vi "Generate multi-line AO sequence.vi"(11 "Variables":T1 {"Dwell time" format="%#_6f"; "Sample Clock Rate" format="%#_6f"}) -> (3 "Pockels modulation sequence":dbl[](array[numeric]))   [LabVIEW 2017]
uses:
  Typedefs/Pockels mod gen variables cluster.ctl
  Typedefs/Imaging Protocols enum.ctl
panel:
  out "Single line (points)":i32
  out "Full sequence (points)":i32
  out "Length of single line (ms)":dbl format="%#_6f"
  out "Length of sequence (ms)":dbl format="%#_6f"
  out "Multi-line pockels modulation waveform":dbl[](graph)
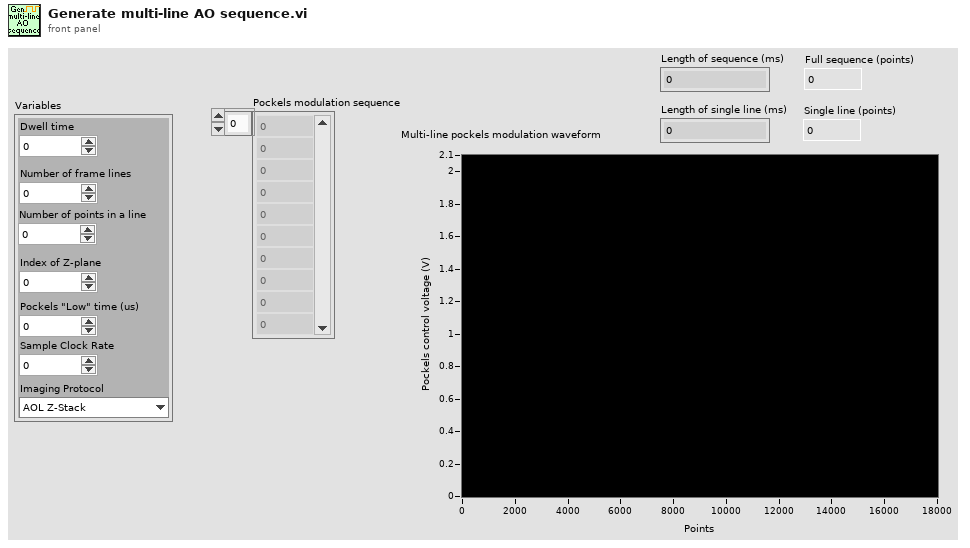
[diagram p1: front panel]
types:
  T1 = typedef "Pockels mod gen variables cluster.ctl" = cluster{"Dwell time":dbl, "Number of frame lines":i32, "Number of points in a line":i32, "Index of Z-plane":i32, "Pockels \"Low\" time (us)":dbl, "Sample Clock Rate":dbl, "Imaging Protocol":T2}
  T2 = typedef "Imaging Protocols enum.ctl" = enum16{"AOL Z-Stack", "Motor Z Stack", "Functional Acquisition", "Single Plane Acquisition", "Volume Acquisition", "Live Imaging", "Live Plane Imaging", "Live Volume Imaging"}
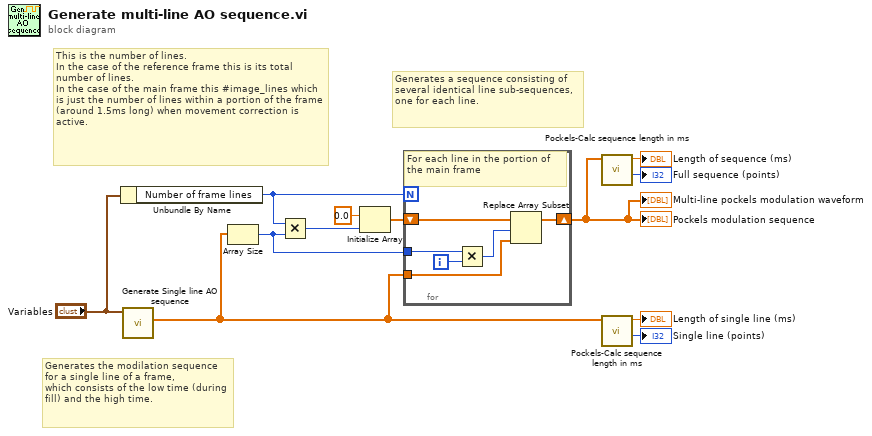
[diagram p0: block diagram]
diagram:
  # "This is the number of lines.\nIn the case of the reference frame this is its total number of lines.\nIn the case of the main frame this #image_lines which is just the number of lines within a portion of the frame (around 1.5ms long) when movement correction is active."
  # "Generates a sequence consisting of several identical line sub-sequences, one for each line."
  # "Generates the modilation sequence for a single line of a frame,\nwhich consists of the low time (during fill) and the high time."
  n1 = Unbundle By Name("Variables") -> ("Number of frame lines"=w8:i32)
  n2 = call "Generate Single line AO sequence.vi"("Variables"="Variables") -> ("Single line AO sequence"=w4:dbl[])  [unwired: 10 in]
  n3 = Array Size(array=w4) -> (size(s)=w12:i32)
  n4 = Multiply(x=w8, y=w12) -> (x*y=w9:i32)
  n5 = Initialize Array(0.0 ("Pockels Value (minimum prevented)"), w9) -> (w11:dbl[])
  n6 = for {
    N: w8 -> [_]
    tunnel: w4 -> [w13]
    shift-right: [w17] -> w3
    shift-left: w11 -> [w18]
    tunnel: w12 -> [w15]
    i -> [w16]
    # "For each line in the portion of the main frame"
    n7 = Multiply(x=w15, y=w16) -> (x*y=w14:i32)
    n8 = Replace Array Subset(array=w18, new element=w13, index=w14) -> (w17:dbl[])
  }
  "Pockels modulation sequence" <- w3
  "Multi-line pockels modulation waveform" <- w3
  n9 = call "Pockels-Calc sequence length in ms.vi"("Pockels modulation sequence in"=w3) -> ("Sequence length (points)"=→"Full sequence (points)":i32, "Sequence length (ms)"=→"Length of sequence (ms)":dbl)  [unwired: 8 in, 1 out]
  n10 = call "Pockels-Calc sequence length in ms.vi"("Pockels modulation sequence in"=w4) -> ("Sequence length (points)"=→"Single line (points)":i32, "Sequence length (ms)"=→"Length of single line (ms)":dbl)  [unwired: 8 in, 1 out]
